vi "Set Display A.vi"(8 "error in (no error)":errorcluster, 9 "function A (z/y:0)":i16(slide)=1 scale=0.0..3.0, 11 "VISA resource name":refnum<visa-resource-name>) -> (0 "error out 2":errorcluster)   [LabVIEW 2017, in "HP4192 Impedance Analyzer.lvlib"]
uses:
  HP4192 Impedance Analyzer.lvlib
panel:
  out "VISA resource name out 2":refnum<visa-resource-name>
  out "error out":errorcluster
  out "VISA resource name out":refnum<visa-resource-name>
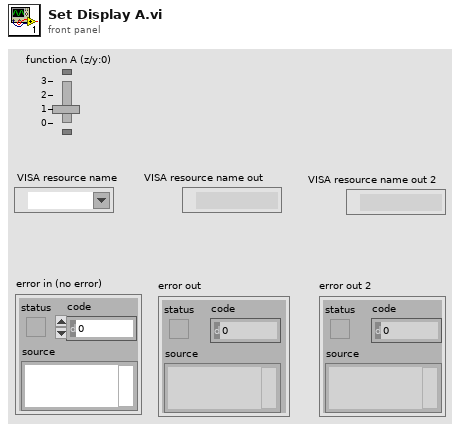
[diagram p1: front panel]
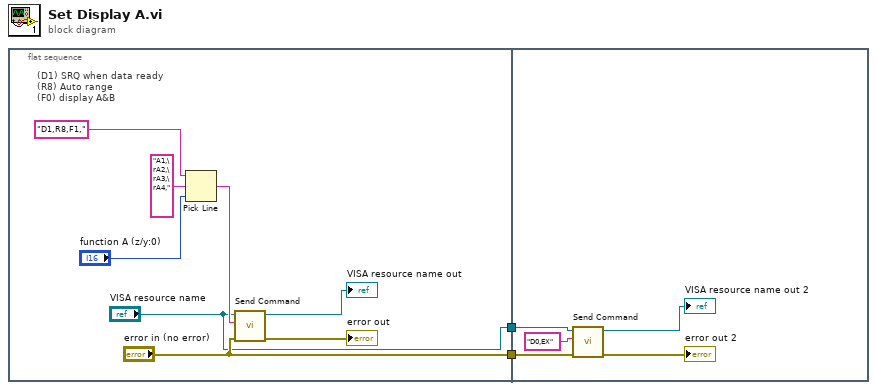
[diagram p0: block diagram]
diagram:
  n1 = flat-sequence {
    tunnel: ["error in (no error)"] -> w2
    tunnel: ["VISA resource name"] -> w1
    tunnel: w2 -> [w12]
    tunnel: w1 -> [w11]
    frame #0 {
      # "(D1) SRQ when data ready\n(R8) Auto range\n(F0) display A&B"
      n2 = Pick Line(string ("")="D1,R8,F1,", multi-line string="A1,\rA2,\rA3,\rA4,", line index="function A (z/y:0)") -> (output string=w5:string)
      n3 = call "Send Command.vi"("error in (no error)"="error in (no error)", "write buffer"=w5, "VISA resource name"="VISA resource name") -> ("error out"=→"error out":errorcluster, "VISA resource name out"=→"VISA resource name out":refnum<visa-resource-name>)  [unwired: 7 in]
    }
    frame #1 {
      n4 = call "Send Command.vi"("error in (no error)"=w12, "write buffer"="D0,EX", "VISA resource name"=w11) -> ("error out"=→"error out 2":errorcluster, "VISA resource name out"=→"VISA resource name out 2":refnum<visa-resource-name>)  [unwired: 7 in]
    }
  }
